vi "6332B输出控制.vi"(8 "错误输入":errorcluster, 10 "Choose Channel":T1={"Channel1"=TRUE, "Channel2"=TRUE, "Channel3"=FALSE}, 11 "VISA资源名称":refnum<visa-resource-name>) -> (0 "错误输出":errorcluster, 3 "VISA资源名称输出":refnum<visa-resource-name>)   [LabVIEW 2020]
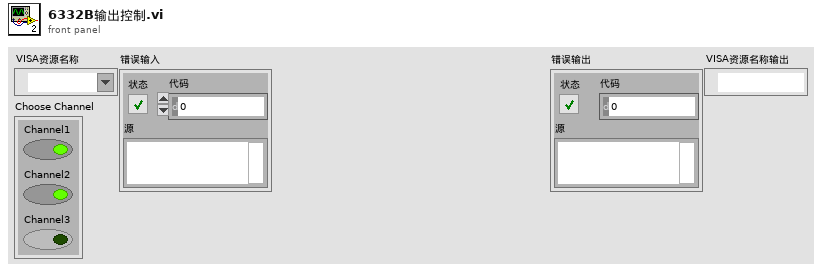
[diagram p1: front panel]
types:
  T1 = cluster{"Channel1":bool, "Channel2":bool, "Channel3":bool}
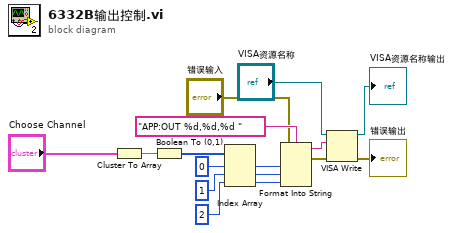
[diagram p0: block diagram]
diagram:
  n1 = Cluster To Array(cluster="Choose Channel") -> (array=w13:bool[])
  n2 = Boolean To (0,1)(Boolean=w13) -> (0, 1=w12:i16[])
  n3 = Index Array(array=w12, index #1=0 ("索引"), index #2=1 ("索引"), index #3=2 ("索引")) -> (element #1=w8:i16, element #2=w7:i16, element #3=w6:i16)
  n4 = Format Into String(format string="APP:OUT %d,%d,%d " ("写入缓冲区"), error in="错误输入", w8, w7, w6) -> (resulting string=w5:string, error out=w4:errorcluster)  [unwired: 1 in]
  n5 = VISA Write(VISA resource name="VISA资源名称", write buffer=w5, error in (no error)=w4) -> (VISA resource name out=→"VISA资源名称输出":refnum<visa-resource-name>, error out=→"错误输出":errorcluster)  [unwired: 1 out]
